vi "XIPIN_SPI-4.2_13_0.vi"   [LabVIEW 2017]
doc: "The Xilinx(R) SPI-4.2 core provides a compliant Packet-Over-SONET/SDH (POS) solution, which can be quickly integrated into networking systems. Through user-configurable options, the SPI-4.2 core provides design flexibility while seamlessly interoperating with industry leading Application Specific Standard Products (ASSPs) to maximize the data transfer bandwidth. The Xilinx SPI-4.2 core is fully compliant with the Optical Internetworking Forum's System Packet Interface Level 4 (SPI-4) Phase 2 standard (OIF-SPI4-02.1), as well as the SATURN(R) Development Group's POS-PHY Level 4 (PL4) interface specification. The PL4 core interfaces between Physical (PHY) and Link layer devices within networking applications, and supports static or dynamic alignment configurations. Dynamic alignment compensates for variations in data path length, allowing the use of multiple connectors and backplanes. The core communicates between devices, using the SPI4.2 interface standard at more than 1-Gbps, enabling OC-192 POS, ATM, and 10 Gb/s Ethernet applications. The Xilinx PL4 core has been verified in hardware to interoperate with PHY and NP devices from PMC-Sierra (S/UNI(R)-9953 (PM5390)), Mindspeed (OptiPHY-F10G (M29730)), and Intel (IXF1810x family).\n------------------------------------\n<b>Need License</b> : Yes\n<b>Interface</b> : AXI4 AXI4-Stream"
uses:
  <vilib>/rvi/XilinxIP/XIPIN_XNode/niFpgaXIPIN.xnode
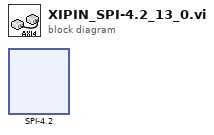
[diagram p0: block diagram]
diagram:
  n1 = xnode ("SPI-4.2")() -> ()
